vi "RT-R45-1.vi"() -> ()   [LabVIEW 2016]
uses:
  <vilib>/FPGAPlugInAG/cRIO-9067/niLvFpga_Open_cRIO-9067.vi
  <vilib>/Utility/error.llb/Error Cluster From Error Code.vi
  <vilib>/rvi/errors/niLvFpgaAdjustHostInterfaceError.vi
  <vilib>/rvi/interface/nirviOpenFPGA/nirviOpenFPGA.xnode
  FPGA Bitfiles/MayUpgrade_FPGA-R45-1_R45-1-FPGA_kkNe-YozHV4.lvbitx
  FPGA-R45-1.vi
  <vilib>/rvi/interface/nirviReadWriteControl/nirviReadWriteControl.xnode
  NiFpgaLv.dll
panel:
  in  "Tab Control":T1(tab)
  out "R45 1 Steerer X":dbl(knob) scale=-10.0..10.0 scale format="%#_4g"
  out "R45 1 Steerer Y":dbl(knob) scale=-10.0..10.0 scale format="%#_4g"
  out "X steerer readbacks":fxp<+/-,27,6> format="%_3g"
  out "Y steerer readbacks":fxp<+/-,27,6> format="%_3g"
  out "R45 Switch magnet faraday cup":bool
  out "R45 Switch magnet Aperture":bool
  out "R-45 FC1 IN":bool
  out "R-45 Aperture 1 IN":bool
  out "Cryo pump":T2
  out "Ion gauge":T3
  out "ig":dbl
  out "cg":dbl
  out "Right Current  monitor":fxp<+/-,26,5>
  out "Right voltage monitor":fxp<+/-,26,5>
  out "Left Current  monitor":fxp<+/-,26,5>
  out "Left voltage monitor":fxp<+/-,26,5>
  out "down Current  monitor":fxp<+/-,26,5>
  out "Down voltage monitor":fxp<+/-,26,5>
  out "Up Current  monitor":fxp<+/-,26,5>
  out "Up voltage monitor":fxp<+/-,26,5>
  out "Right":dbl(knob) scale=0.0..10.0 scale format="%#_4g"
  out "Left":dbl(knob) scale=0.0..10.0 scale format="%#_4g"
  out "Down":dbl(knob) scale=0.0..10.0 scale format="%#_4g"
  out "Up":dbl(knob) scale=0.0..10.0 scale format="%#_4g"
  out "2nd stage":u8[](array[numeric])
  out "1st stage":u8[](array[numeric])
  out "Pump On":u8[](array[numeric])
  out "Time since repurge":u8[](array[numeric])
  out "Ion gauge 1":u8[](array[numeric])
  out "Convectron 1":u8[](array[numeric])
  out "Ion gauge 2":u8[](array[numeric])
  out "Convectron 2":u8[](array[numeric])
  in  "Ion gauge 3":T3
  in  "Cryo pump 2":T2
  out "Vac Cluster error":errorcluster
  out "DIO OUTPUT":bool[](array[boolean])
  in  "Numeric value out":dbl
  out "Numeric value out 2":dbl
  out "Numeric value out 3":dbl
  out "ion gauge interlock 1":bool
  out "CG interlock 1":bool
  out "interlocked tripped":bool
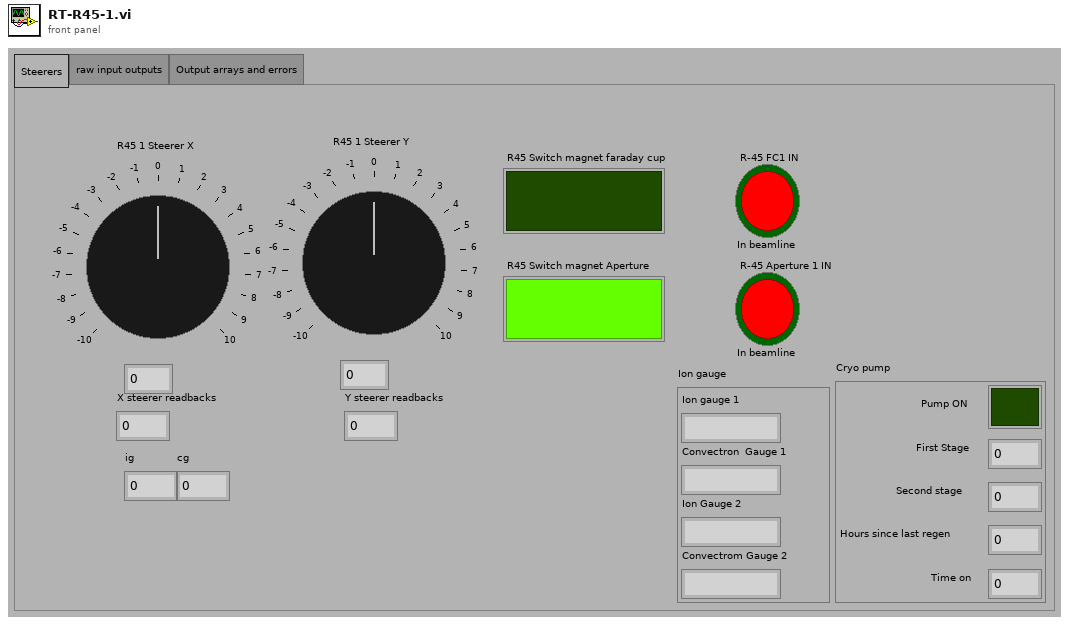
[diagram p1: front panel]
types:
  T1 = enum32{"Steerers", "raw input outputs", "Output arrays and errors"}
  T2 = cluster{"First Stage":dbl, "Second stage":dbl, "Hours since last regen":dbl, "Pump ON":bool, "Time on":dbl}
  T3 = cluster{"Ion gauge 1":string, "Convectron  Gauge 1 ":string, "Ion Gauge 2":string, "Convectrom Gauge 2":string}
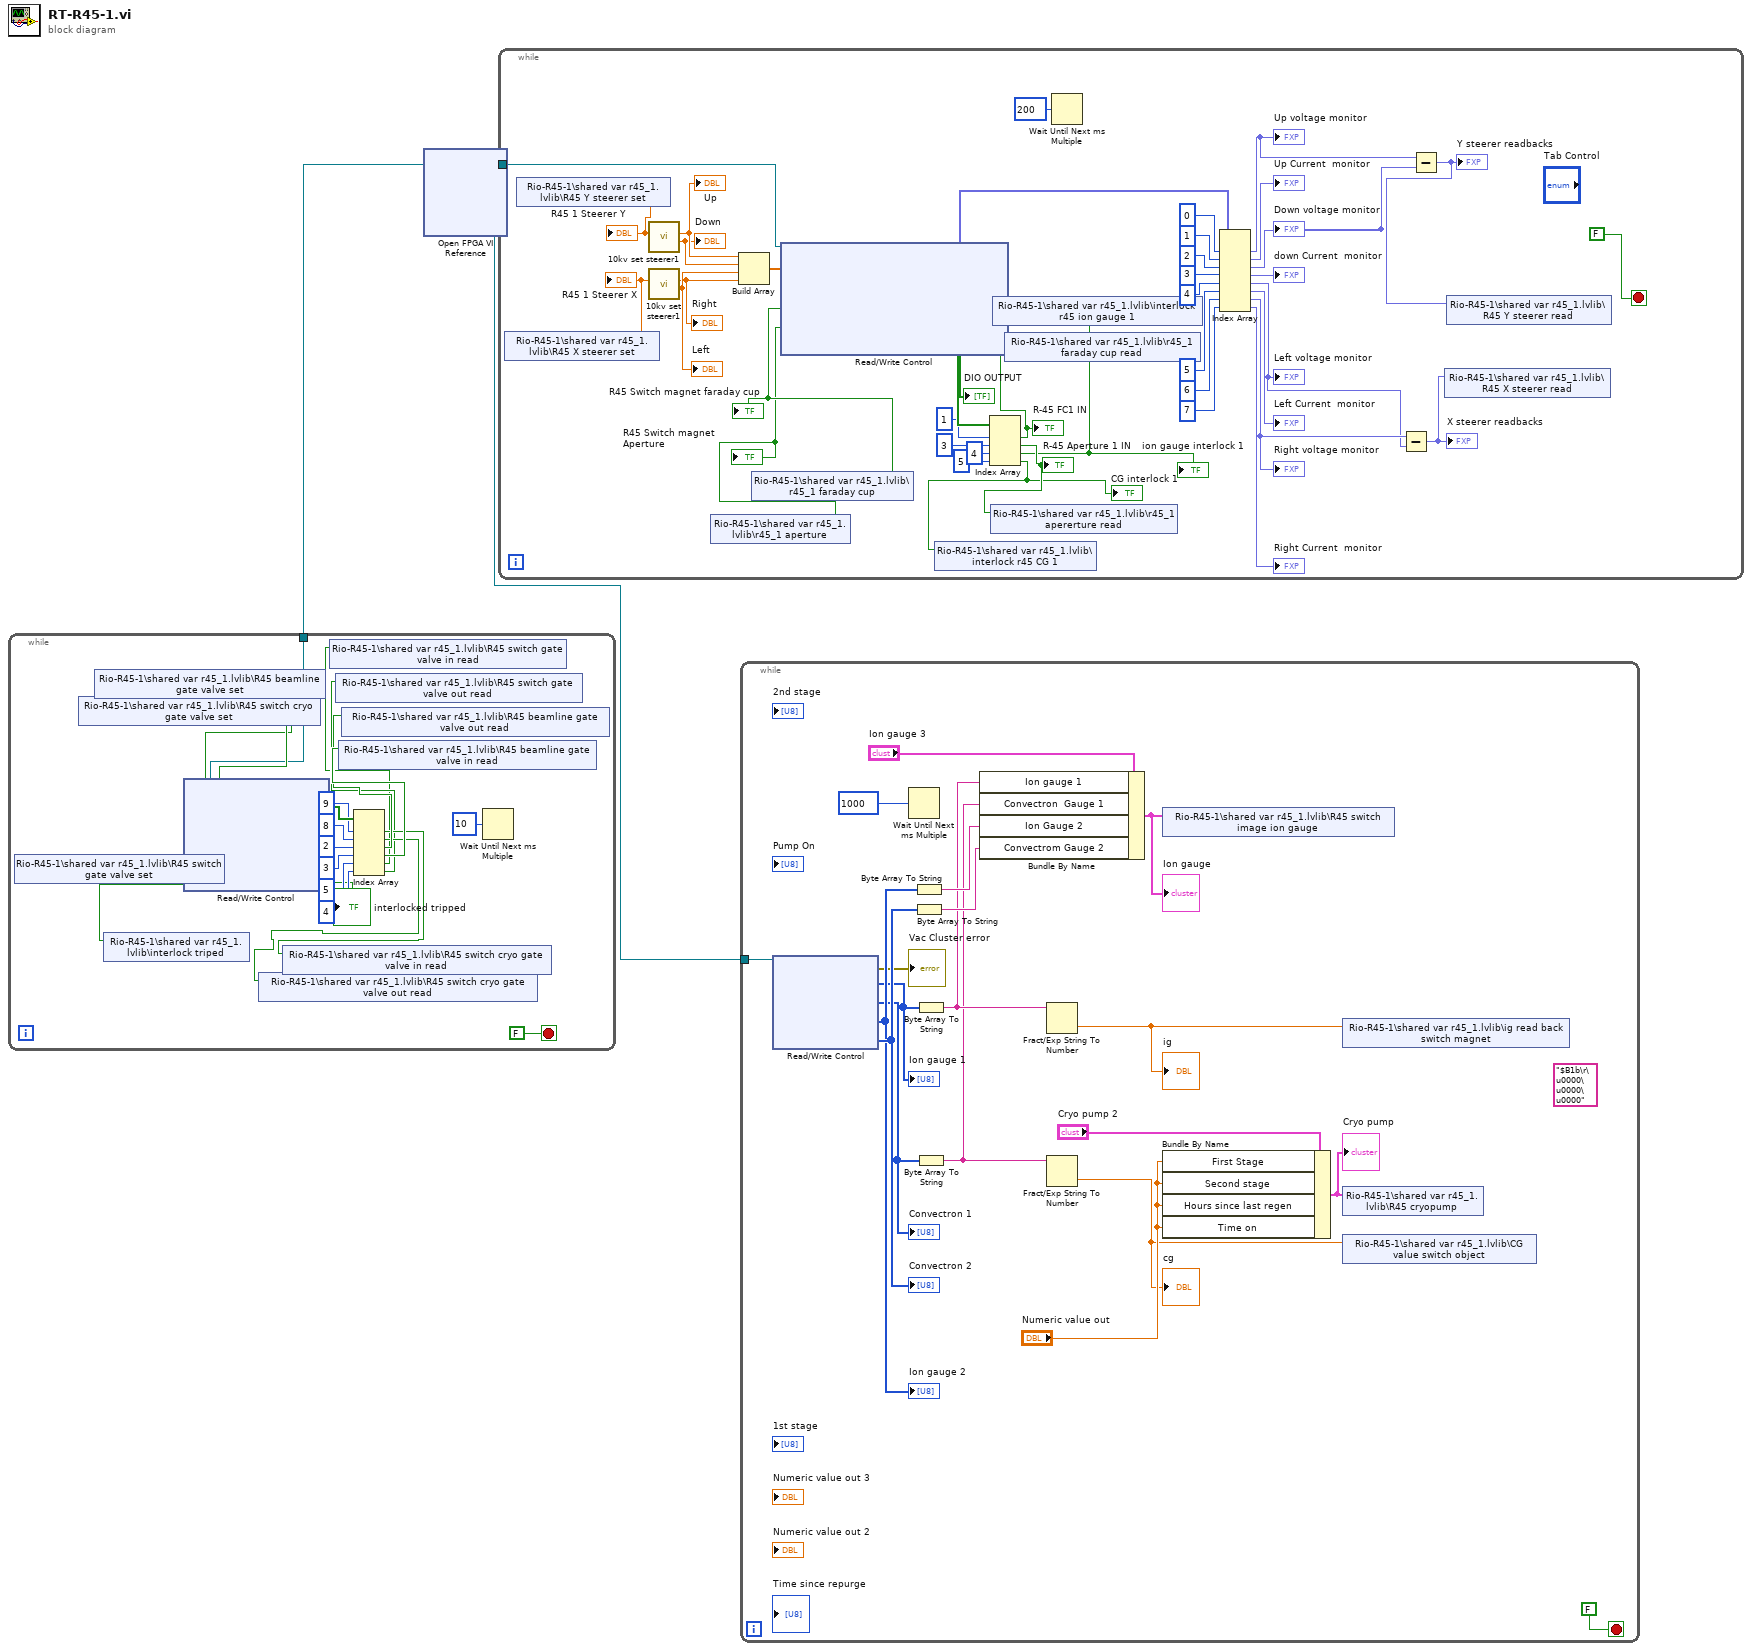
[diagram p0: block diagram]
diagram:
  n1 = xnode "Open FPGA VI Reference"() -> ("FPGA VI Reference Out"=w1:refnum<k20>)  [unwired: 2 in, 1 out]
  n2 = while {
    tunnel: w1 -> [w11]
    stop <- FALSE stop-if-true
    n3 = shared-variable "Rio-R45-1\\shared var r45_1.lvlib\\R45 switch gate valve set"() -> (w8:bool)  [unwired: 1 in, 1 out]
    n4 = shared-variable "Rio-R45-1\\shared var r45_1.lvlib\\R45 switch cryo gate valve set"() -> (w21:bool)  [unwired: 1 in, 1 out]
    n5 = shared-variable "Rio-R45-1\\shared var r45_1.lvlib\\R45 beamline gate valve set"() -> (w7:bool)  [unwired: 1 in, 1 out]
    n6 = xnode "Read/Write Control"("FPGA VI Reference In"=w11, "Mod8/CH3"=w8, "Mod8/CH4"=w21, "Mod8/CH2"=w7) -> ("DI Gate Valves"=w20:bool[], "interlocked tripped"=w2:bool)  [unwired: 1 in, 2 out]
    "interlocked tripped" <- w2
    n7 = shared-variable "Rio-R45-1\\shared var r45_1.lvlib\\interlock triped"(w2) -> ()  [unwired: 1 in, 1 out]
    n8 = Index Array(array=w20, index #1=9 ("index"), index #2=8 ("index"), index #3=2 ("index"), index #4=3 ("index"), index #5=5 ("index"), index #6=4 ("index")) -> (element #1=w6:bool, element #2=w5:bool, element #3=w12:bool, element #4=w13:bool, element #5=w3:bool, element #6=w4:bool)
    n9 = shared-variable "Rio-R45-1\\shared var r45_1.lvlib\\R45 switch cryo gate valve out read"(w5) -> ()  [unwired: 1 in, 1 out]
    n10 = shared-variable "Rio-R45-1\\shared var r45_1.lvlib\\R45 switch cryo gate valve in read"(w6) -> ()  [unwired: 1 in, 1 out]
    n11 = shared-variable "Rio-R45-1\\shared var r45_1.lvlib\\R45 switch gate valve in read"(w3) -> ()  [unwired: 1 in, 1 out]
    n12 = shared-variable "Rio-R45-1\\shared var r45_1.lvlib\\R45 switch gate valve out read"(w4) -> ()  [unwired: 1 in, 1 out]
    n13 = shared-variable "Rio-R45-1\\shared var r45_1.lvlib\\R45 beamline gate valve in read"(w13) -> ()  [unwired: 1 in, 1 out]
    n14 = shared-variable "Rio-R45-1\\shared var r45_1.lvlib\\R45 beamline gate valve out read"(w12) -> ()  [unwired: 1 in, 1 out]
    n15 = Wait Until Next ms Multiple(millisecond multiple=u32 10) -> ()  [unwired: 1 out]
  }
  n16 = while {
    tunnel: w1 -> [w61]
    stop <- FALSE stop-if-true
    n17 = shared-variable "Rio-R45-1\\shared var r45_1.lvlib\\R45 X steerer set"() -> (w32:dbl)  [unwired: 1 in, 1 out]
    "R45 1 Steerer X" <- w32
    n18 = shared-variable "Rio-R45-1\\shared var r45_1.lvlib\\R45 Y steerer set"() -> (w33:dbl)  [unwired: 1 in, 1 out]
    "R45 1 Steerer Y" <- w33
    n19 = call "10kv set steerer1.vi"("Steerer Control IN"=w33) -> ("- Steerer"=w40:dbl, "+ Steerer"=w41:dbl)  [unwired: 8 in, 1 out]
    "Down" <- w40
    "Up" <- w41
    n20 = call "10kv set steerer1.vi"("Steerer Control IN"=w32) -> ("- Steerer"=w39:dbl, "+ Steerer"=w38:dbl)  [unwired: 8 in, 1 out]
    "Left" <- w39
    "Right" <- w38
    n21 = shared-variable "Rio-R45-1\\shared var r45_1.lvlib\\r45_1 aperture"() -> (w26:bool)  [unwired: 1 in, 1 out]
    "R45 Switch magnet Aperture" <- w26
    n22 = Build Array(w41, w40, w39, w38) -> (w60:dbl[])
    n23 = shared-variable "Rio-R45-1\\shared var r45_1.lvlib\\r45_1 faraday cup"() -> (w27:bool)  [unwired: 1 in, 1 out]
    "R45 Switch magnet faraday cup" <- w27
    n24 = xnode "Read/Write Control"("FPGA VI Reference In"=w61, "Analog Output"=w60, "R45 Switch magnet faraday cup"=w27, "R45 Switch magnet Aperture"=w26) -> ("Analog input"=w59:fxp<+/-,26,5>[], "DIO OUTPUT"=w45:bool[])  [unwired: 1 in, 2 out]
    "DIO OUTPUT" <- w45
    n25 = Index Array(array=w45, index #1=1 ("index"), index #2=3 ("index"), index #3=4 ("index"), index #4=5 ("index")) -> (element #1=w29:bool, element #2=w28:bool, element #3=w22:bool, element #4=w23:bool)
    "R-45 FC1 IN" <- w29
    "R-45 Aperture 1 IN" <- w28
    "ion gauge interlock 1" <- w22
    "CG interlock 1" <- w23
    n26 = shared-variable "Rio-R45-1\\shared var r45_1.lvlib\\interlock r45 CG 1"(w23) -> ()  [unwired: 1 in, 1 out]
    n27 = shared-variable "Rio-R45-1\\shared var r45_1.lvlib\\r45_1 apererture read"(w28) -> ()  [unwired: 1 in, 1 out]
    n28 = shared-variable "Rio-R45-1\\shared var r45_1.lvlib\\interlock r45 ion gauge 1"(w22) -> ()  [unwired: 1 in, 1 out]
    n29 = shared-variable "Rio-R45-1\\shared var r45_1.lvlib\\r45_1 faraday cup read"(w29) -> ()  [unwired: 1 in, 1 out]
    n30 = Wait Until Next ms Multiple(millisecond multiple=u32 200) -> ()  [unwired: 1 out]
    n31 = Index Array(array=w59, index #1=0 ("index"), index #2=1 ("index"), index #3=2 ("index"), index #4=3 ("index"), index #5=4 ("index"), index #6=5 ("index"), index #7=6 ("index"), index #8=7 ("index")) -> (element #1=w37:fxp<+/-,26,5>, element #2=→"Up Current  monitor":fxp<+/-,26,5>, element #3=w36:fxp<+/-,26,5>, element #4=→"down Current  monitor":fxp<+/-,26,5>, element #5=w34:fxp<+/-,26,5>, element #6=→"Left Current  monitor":fxp<+/-,26,5>, element #7=w35:fxp<+/-,26,5>, element #8=→"Right Current  monitor":fxp<+/-,26,5>)
    "Up voltage monitor" <- w37
    "Down voltage monitor" <- w36
    "Left voltage monitor" <- w34
    "Right voltage monitor" <- w35
    n32 = Subtract(x=w35, y=w34) -> (x-y=w30:fxp<+/-,27,6>)
    "X steerer readbacks" <- w30
    n33 = Subtract(x=w37, y=w36) -> (x-y=w31:fxp<+/-,27,6>)
    "Y steerer readbacks" <- w31
    n34 = shared-variable "Rio-R45-1\\shared var r45_1.lvlib\\R45 X steerer read"(w30) -> ()  [unwired: 1 in, 1 out]
    n35 = shared-variable "Rio-R45-1\\shared var r45_1.lvlib\\R45 Y steerer read"(w31) -> ()  [unwired: 1 in, 1 out]
  }
  n36 = while {
    tunnel: w1 -> [w72]
    stop <- FALSE stop-if-true
    (unwired) "$B1b\r\u0000\u0000\u0000" ("string 2")
    n37 = xnode "Read/Write Control"("FPGA VI Reference In"=w72) -> ("error out"=→"Vac Cluster error":errorcluster, "Ion gauge 1"=w75:u8[], "Convectron 1"=w65:u8[], "Ion gauge 2"=w76:u8[], "Convectron 2"=w77:u8[])  [unwired: 1 in, 1 out]
    "Ion gauge 1" <- w75
    "Convectron 1" <- w65
    "Ion gauge 2" <- w76
    "Convectron 2" <- w77
    n38 = Wait Until Next ms Multiple(millisecond multiple=u32 1000) -> ()  [unwired: 1 out]
    n39 = Byte Array To String(unsigned byte array=w76) -> (string=w78:string)
    n40 = Byte Array To String(unsigned byte array=w77) -> (string=w79:string)
    n41 = Byte Array To String(unsigned byte array=w75) -> (string=w66:string)
    n42 = Byte Array To String(unsigned byte array=w65) -> (string=w64:string)
    n43 = Bundle By Name(cluster="Ion gauge 3", "Ion gauge 1"=w66, "Convectron  Gauge 1"=w64, "Ion Gauge 2"=w78, "Convectrom Gauge 2"=w79) -> (w69:T3)
    "Ion gauge" <- w69
    n44 = Fract/Exp String To Number(string=w66) -> (number=w63:dbl)  [unwired: 3 in, 1 out]
    "ig" <- w63
    n45 = Fract/Exp String To Number(string=w64) -> (number=w62:dbl)  [unwired: 3 in, 1 out]
    "cg" <- w62
    n46 = shared-variable "Rio-R45-1\\shared var r45_1.lvlib\\R45 switch image ion gauge"(w69) -> ()  [unwired: 1 in, 1 out]
    n47 = Bundle By Name(cluster="Cryo pump 2", "First Stage"="Numeric value out", "Second stage"="Numeric value out", "Hours since last regen"="Numeric value out", "Time on"="Numeric value out") -> (w68:T2)
    "Cryo pump" <- w68
    n48 = shared-variable "Rio-R45-1\\shared var r45_1.lvlib\\ig read back switch magnet"(w63) -> ()  [unwired: 1 in, 1 out]
    n49 = shared-variable "Rio-R45-1\\shared var r45_1.lvlib\\R45 cryopump"(w68) -> ()  [unwired: 1 in, 1 out]
    n50 = shared-variable "Rio-R45-1\\shared var r45_1.lvlib\\CG value switch object"(w62) -> ()  [unwired: 1 in, 1 out]
  }
